vi "GetAllData.vi"(8 "error in (no error)":errorcluster, 10 "handle in":i32) -> (0 "error out":errorcluster, 2 "handle out":i32, 3 "Data cluster":T1)   [LabVIEW 2014]
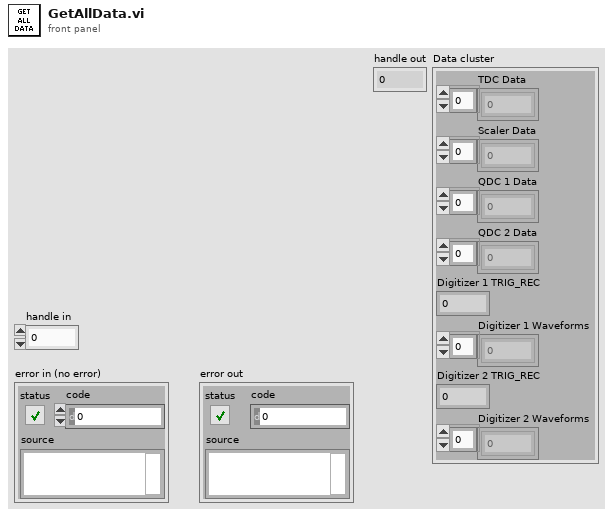
[diagram p1: front panel]
types:
  T1 = cluster{"TDC Data":u32[], "Scaler Data":u32[], "QDC 1 Data":u32[], "QDC 2 Data":u32[], "Digitizer 1 TRIG_REC":u32, "Digitizer 1 Waveforms":u32[], "Digitizer 2 TRIG_REC":u32, "Digitizer 2 Waveforms":u32[]}
  T2 = cluster{"TDC":u32, "Scaler":u32, "QDC 1":u32, "QDC 2":u32, "Digitizer 1":u32, "Digitizer 2":u32}
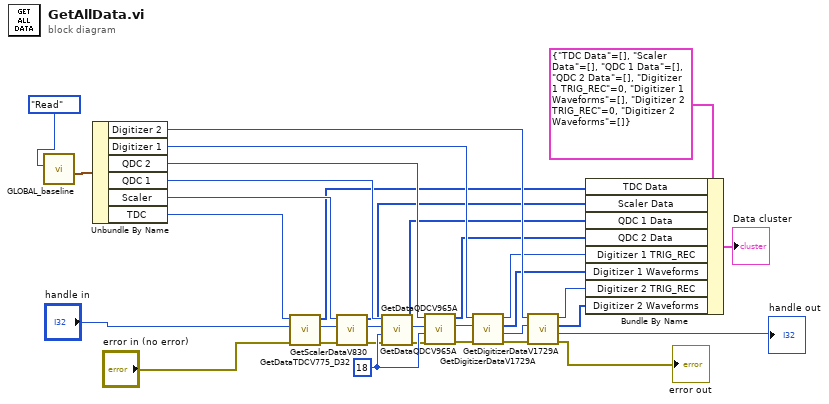
[diagram p0: block diagram]
diagram:
  w33 = 18 ("#samples")
  n1 = call "GLOBAL_baseline.vi"("State"=enum16{"Initialise", "Write", "Read"}."Read") -> ("Addresses Out"=w23:T2)  [unwired: 10 in]
  n2 = Unbundle By Name(w23) -> ("Digitizer 2"=w13:u32, "Digitizer 1"=w16:u32, "QDC 2"=w19:u32, "QDC 1"=w20:u32, "Scaler"=w21:u32, "TDC"=w22:u32)
  n3 = call "GetDataTDCV775_D32.vi"("error in (no error)"="error in (no error)", "handle in"="handle in", "VME Base Address"=w22) -> ("error out"=w27:errorcluster, "handle out"=w28:i32, "Array"=w10:u32[])  [unwired: 6 in]
  n4 = call "GetScalerDataV830.vi"("error in (no error)"=w27, "handle in"=w28, "VME Base Address"=w21) -> ("error out"=w29:errorcluster, "handle out"=w30:i32, "Buff"=w9:u32[])  [unwired: 6 in]
  n5 = call "GetDataQDCV965A.vi"("error in (no error)"=w29, "#samples"=w33, "handle in"=w30, "VME module Base Address"=w20) -> ("error out"=w31:errorcluster, "handle out"=w32:i32, "Data"=w8:u32[])  [unwired: 5 in]
  n6 = call "GetDataQDCV965A.vi"("error in (no error)"=w31, "#samples"=w33, "handle in"=w32, "VME module Base Address"=w19) -> ("error out"=w18:errorcluster, "handle out"=w17:i32, "Data"=w7:u32[])  [unwired: 5 in]
  n7 = call "GetDigitizerDataV1729A.vi"("error in (no error)"=w18, "handle in"=w17, "VME Base Address"=w16) -> ("error out"=w15:errorcluster, "handle out"=w14:i32, "Waveform"=w5:u32[], "TRIG_REC"=w6:u32)  [unwired: 5 in]
  n8 = call "GetDigitizerDataV1729A.vi"("error in (no error)"=w15, "handle in"=w14, "VME Base Address"=w13) -> ("error out"=→"error out":errorcluster, "handle out"=→"handle out":i32, "Waveform"=w3:u32[], "TRIG_REC"=w4:u32)  [unwired: 5 in]
  n9 = Bundle By Name(cluster=T1 {"TDC Data"=[], "Scaler Data"=[], "QDC 1 Data"=[], "QDC 2 Data"=[], "Digitizer 1 TRIG_REC"=0, "Digitizer 1 Waveforms"=[], "Digitizer 2 TRIG_REC"=0, "Digitizer 2 Waveforms"=[]}, "TDC Data"=w10, "Scaler Data"=w9, "QDC 1 Data"=w8, "QDC 2 Data"=w7, "Digitizer 1 TRIG_REC"=w6, "Digitizer 1 Waveforms"=w5, "Digitizer 2 TRIG_REC"=w4, "Digitizer 2 Waveforms"=w3) -> (→"Data cluster":T1)
